vi "HTS Front Panel.vi"() -> ()   [LabVIEW 2019, in "Results.lvlib" / "Water Tunnel Results.lvclass"]
uses:
  Water Tunnel Results.lvclass
  Test Stands/HTS/HTS Test Stand.lvclass
panel:
  out "Adjusted":bool
  in  "Htr Temp SP":dbl=292.0 caption="Heater Temperature" min=0.0 max=372.0 step=1.0
  in  "auto Temp":bool
  in  "Htr MOS Ctrl":dbl caption="Heater MOS Control" min=0.0 max=10.0 step=0.1
  in  "Htr Pwr SP":dbl caption="Heater Power" min=0.0 max=300.0 step=1.0
  out "Heater Power":dbl(slide) scale=0.0..100.0
  in  "auto pwr":bool
  out "Heater dU":dbl format="%#.3f"
  out "Shunt dU":dbl format="%#.4f"
  out "aslant":dbl format="%#.2f"
  out "outer":dbl format="%#.2f"
  out "inner":dbl format="%#.2f"
  out "above":dbl format="%#.2f"
  out "inside":dbl format="%#.2f"
  out "I":dbl format="%#.3f"
  out "P":dbl format="%#.3f"
  out "Data":waveform(dbl)[](graph) caption="Temperatures"
  # "Automatic"
  # "A"
  # "W"
  # "Manual"
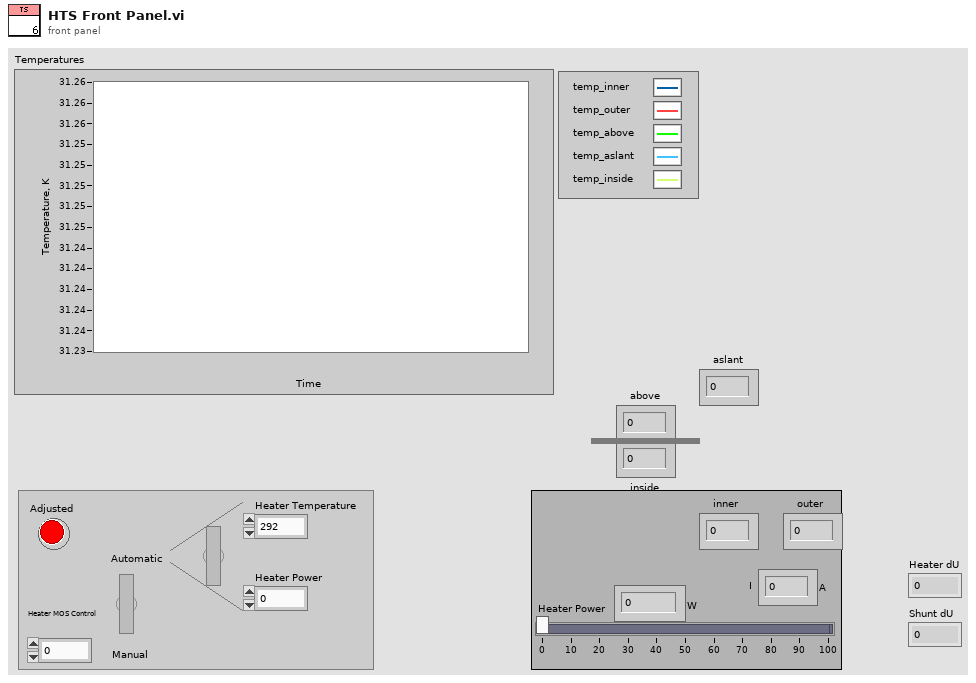
[diagram p1: front panel]
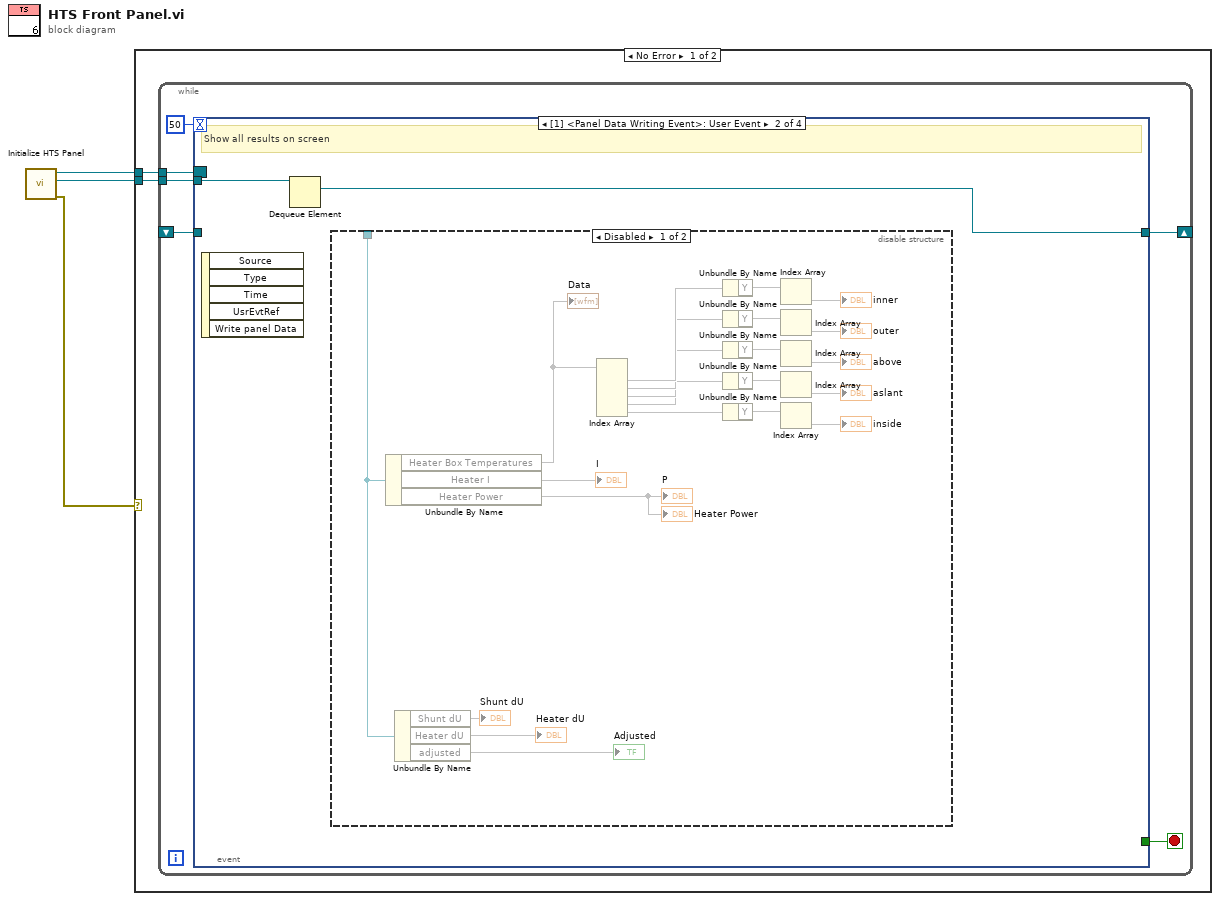
[diagram p0: block diagram]
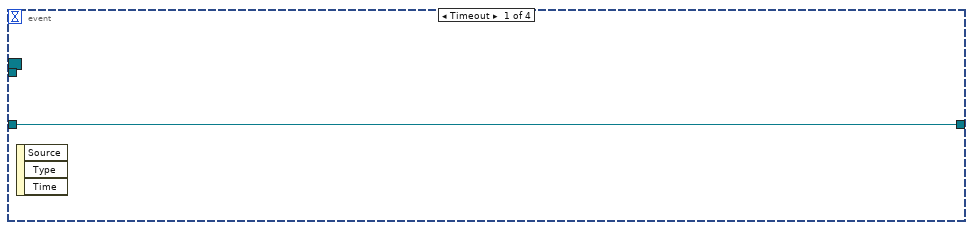
[diagram p2: hidden frame]
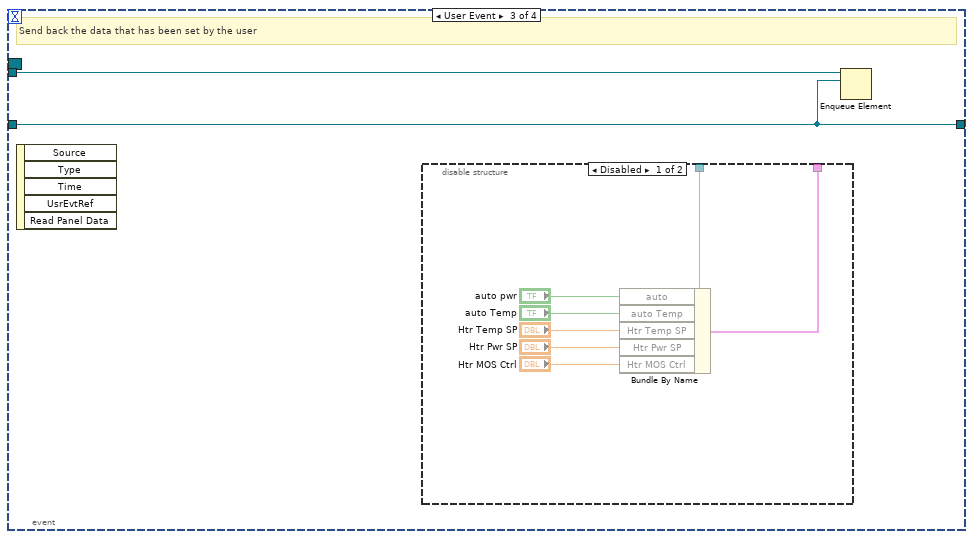
[diagram p4: hidden frame]
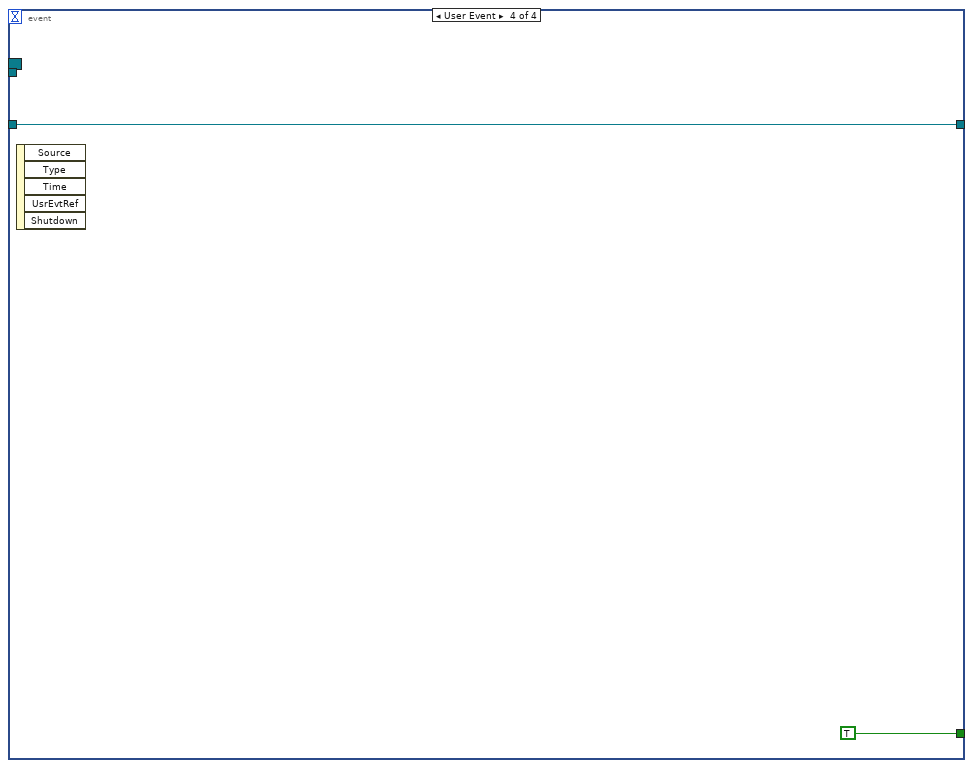
[diagram p6: hidden frame]
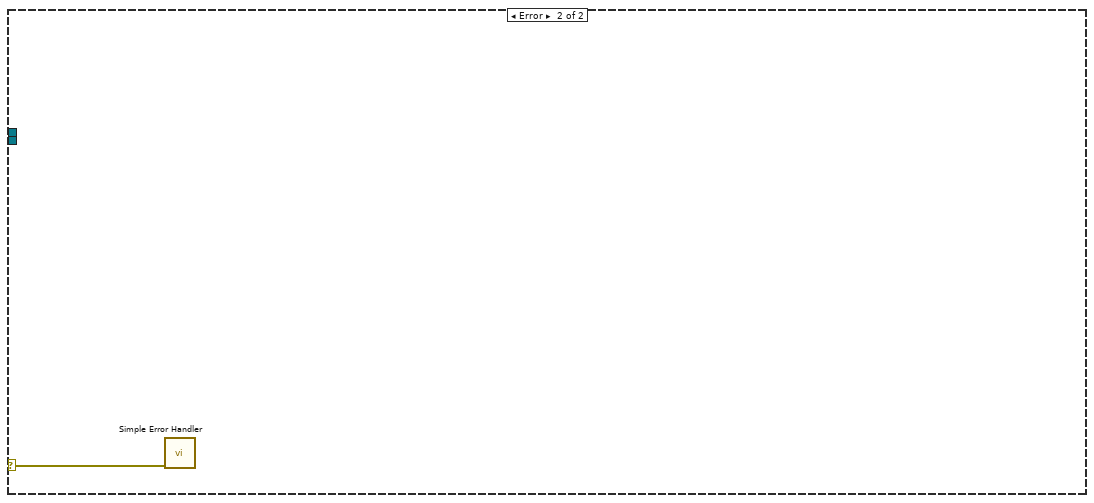
[diagram p7: hidden frame]
diagram:
  n1 = call "Initialize HTS Panel.vi"() -> ("error out"=w2:errorcluster, "HTS Results queue out"=w1:refnum<queue>, "Event Registration Refnum"=w3:refnum<event-registration>)  [unwired: 9 in]
  n2 = case shown="No Error" w2 {
    selector: w2 -> [_ w48]
    tunnel: w3 -> [w5 _]
    tunnel: w1 -> [w4 _]
    frame No Error {
      n3 = while {
        tunnel: w5 -> [w10]
        tunnel: w4 -> [w9]
        shift-right: [w7] -> _
        shift-left: _ -> [w6]
        stop <- w11 stop-if-true
        n4 = event shown="[1] <Panel Data Writing Event>: User Event" {
          selector: w10 -> [_ _ _ _]
          dyn-events: _ -> [_ _ _ _]
          timeout: 50 -> [_ _ _ _]
          tunnel: [_ _ _ TRUE] -> w11
          tunnel: w9 -> [_ w14 w38 _]
          tunnel: [w12 w13 w37 w46] -> w7
          tunnel: w6 -> [w12 _ w37 w46]
          event Timeout {
            n5 = event-data() -> ()  [unwired: 1 in, 3 out]
          }
          event User Event {
            # "Show all results on screen"
            n6 = event-data() -> ()  [unwired: 1 in, 5 out]
            n7 = Dequeue Element(queue=w14) -> (element=w13:refnum<class "HTS Results.lvclass">)  [unwired: 2 in, 3 out]
            n8 = disable-structure shown="Disabled" {
              disable-tunnel: _ -> [w19 _]
              frame Disabled {
                n9 = Unbundle By Name(w19) -> ("Heater Box Temperatures"=w36, "Heater I"=→"I", "Heater Power"=→"P" →"Heater Power")
                "Data" <- w36
                n10 = Unbundle By Name(w19) -> ("Shunt dU"=→"Shunt dU", "Heater dU"=→"Heater dU", "adjusted"=→"Adjusted")
                n11 = Index Array(array=w36) -> (element #1=w35, element #2=w32, element #3=w29, element #4=w27, element #5=w25)  [unwired: 5 in]
                n12 = Unbundle By Name(w35) -> ("Y"=w34)
                n13 = Unbundle By Name(w32) -> ("Y"=w31)
                n14 = Unbundle By Name(w29) -> ("Y"=w28)
                n15 = Unbundle By Name(w27) -> ("Y"=w26)
                n16 = Unbundle By Name(w25) -> ("Y"=w24)
                n17 = Index Array(array=w34) -> (element=→"inner")  [unwired: 1 in]
                n18 = Index Array(array=w31) -> (element=→"outer")  [unwired: 1 in]
                n19 = Index Array(array=w28) -> (element=→"above")  [unwired: 1 in]
                n20 = Index Array(array=w26) -> (element=→"aslant")  [unwired: 1 in]
                n21 = Index Array(array=w24) -> (element=→"inside")  [unwired: 1 in]
              }
              frame Enabled {
              }
            }
          }
          event User Event {
            # "Send back the data that has been set by the user"
            n22 = event-data() -> ()  [unwired: 1 in, 5 out]
            n23 = disable-structure shown="Disabled" {
              disable-tunnel: _ -> [w45 _]
              disable-tunnel: [w44 _] -> _
              frame Disabled {
                n24 = Bundle By Name(cluster=w45, "auto"="auto pwr", "auto Temp"="auto Temp", "Htr Temp SP"="Htr Temp SP", "Htr Pwr SP"="Htr Pwr SP", "Htr MOS Ctrl"="Htr MOS Ctrl") -> (w44:cluster{})
              }
              frame Enabled {
              }
            }
            n25 = Enqueue Element(queue=w38, element=w37) -> ()  [unwired: 2 in, 3 out]
          }
          event User Event {
            n26 = event-data() -> ()  [unwired: 1 in, 5 out]
          }
        }
      }
    }
    frame Error {
      n27 = call <vilib>:"Simple Error Handler.vi"("error in (no error)"=w48) -> ()  [unwired: 4 in, 5 out]
    }
  }
